vi "integrate.vi"(5 "waiting iterations per pixel":u32, 7 "integration iterations per pixel":u32, 9 "iteration counter in":u32, 10 "sampling values in":T1, 11 "previous pixel values in":T1) -> (1 "finished?":bool, 2 "iteration counter out":u32, 3 "new pixel values out":T1)   [LabVIEW 2010]
uses:
  common_typedefs/channels_cluster.ctl
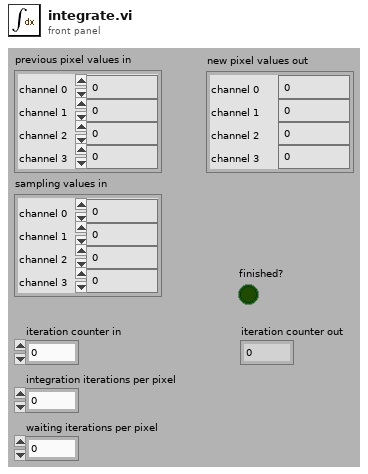
[diagram p1: front panel]
types:
  T1 = typedef "channels_cluster.ctl" = cluster{"channel 0":u32, "channel 1":u32, "channel 2":u32, "channel 3":u32}
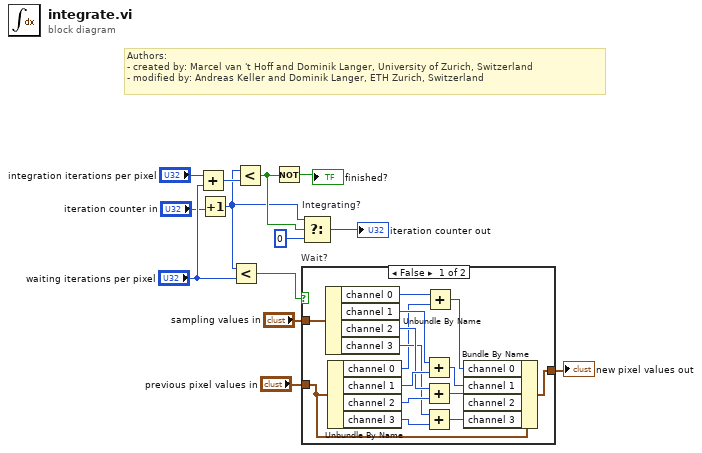
[diagram p0: block diagram]
diagram:
  # "Authors: \n- created by: Marcel van 't Hoff and Dominik Langer, University of Zurich, Switzerland\n- modified by: Andreas Keller and Dominik Langer, ETH Zurich, Switzerland"
  n1 = Add(x="integration iterations per pixel", y="waiting iterations per pixel") -> (x+y=w7:u32)
  n2 = Increment(x="iteration counter in") -> (x+1=w4:u32)
  n3 = Less?(x=w4, y="waiting iterations per pixel") -> (x < y?=w8:bool)
  n4 = Less?(x=w4, y=w7) -> (x < y?=w5:bool)
  n5 = Not(x=w5) -> (.not. x?=→"finished?":bool)
  n6 = Select "Integrating?"(t=w4, s=w5, f=u32 0) -> (s? t:f=→"iteration counter out":u32)
  n7 = case "Wait?" shown="False" w8 {
    tunnel: "sampling values in" -> [w22 _]
    tunnel: "previous pixel values in" -> [w21 w29]
    tunnel: [w16 w29] -> w12
    frame False {
      n8 = Unbundle By Name(w22) -> ("channel 0"=w28:u32, "channel 1"=w27:u32, "channel 2"=w25:u32, "channel 3"=w23:u32)
      n9 = Unbundle By Name(w21) -> ("channel 0"=w14:u32, "channel 1"=w26:u32, "channel 2"=w24:u32, "channel 3"=w15:u32)
      n10 = Add(x=w27, y=w26) -> (x+y=w19:u32)
      n11 = Add(x=w25, y=w24) -> (x+y=w18:u32)
      n12 = Add(x=w23, y=w15) -> (x+y=w17:u32)
      n13 = Add(x=w28, y=w14) -> (x+y=w20:u32)
      n14 = Bundle By Name(cluster=w21, "channel 0"=w20, "channel 1"=w19, "channel 2"=w18, "channel 3"=w17) -> (w16:T1)
    }
    frame True {
    }
  }
  "new pixel values out" <- w12
